vi "Estacionamiento lleno VI.vi"() -> (2 "Retroceder LED":bool)   [LabVIEW 2024]
panel:
  in  "Retroceder":bool
  out "Mensaje":string
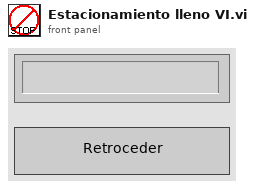
[diagram p1: front panel]
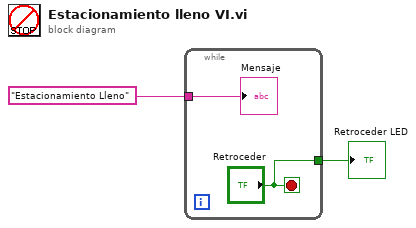
[diagram p0: block diagram]
diagram:
  n1 = while {
    tunnel: "Estacionamiento Lleno" ("Mensaje") -> [w4]
    tunnel: ["Retroceder"] -> w1
    stop <- "Retroceder" stop-if-true
    "Mensaje" <- w4
  }
  "Retroceder LED" <- w1
